vi "Autonomous Independent.vi"   [LabVIEW 2011]
doc: "This VI is called when autonomous begins, and will automatically be terminated when autonomous ends. You can carry out timed or sensor driven robot movement independently without needing to return to the caller."
uses:
  Robot Global Data.vi
types:
  T1 = typedef "WPI_MotorControlDeviceRef.ctl" = cluster{"DeviceStatus":errorcluster, "Type":enum16{"PWM", "CAN"}, "PWM":cluster{"Digital Module":T2, "PWM Channel":T3, "DeadBand":T4}, "CAN":cluster{"Device Number":u8, "Control Mode":T5, "Semaphore":T6, "Max Vout":dbl}, "Invert":bool, "TransformRef":T7, "InvTransformRef":T7}
  T2 = typedef "FPGA_TypedefDigitalModule.ctl" = enum16{"Digital Module 1", "Digital Module 2"}
  T3 = typedef "FPGA_DIOPWMChannel.ctl" = enum8{"PWM 1", "PWM 2", "PWM 3", "PWM 4", "PWM 5", "PWM 6", "PWM 7", "PWM 8", "PWM 9", "PWM 10", "Invalid"}
  T4 = typedef "WPI_PWMDeadband.ctl" = cluster{"Name":string, "maxPositivePwm":i32, "minPositivePwm":i32, "centerPwm":i32, "maxNegativePwm":i32, "minNegativePwm":i32, "angularRange":u16}
  T5 = typedef "WPI_CANJaguar_ControlMode.ctl" = enum8{"Percent VBus", "Current", "Speed", "Position", "Voltage"}
  T6 = typedef "Semaphore RefNum" = refnum<k1>
  T7 = typedef "WPI_PWMTransform_ConPane.ctl" = refnum<vi>
  T8 = typedef "WPI_ServoDeviceRef.ctl" = cluster{"DeviceStatus":errorcluster, "Digital Module":T2, "PWM Channel":T3, "DeadBand":T4}
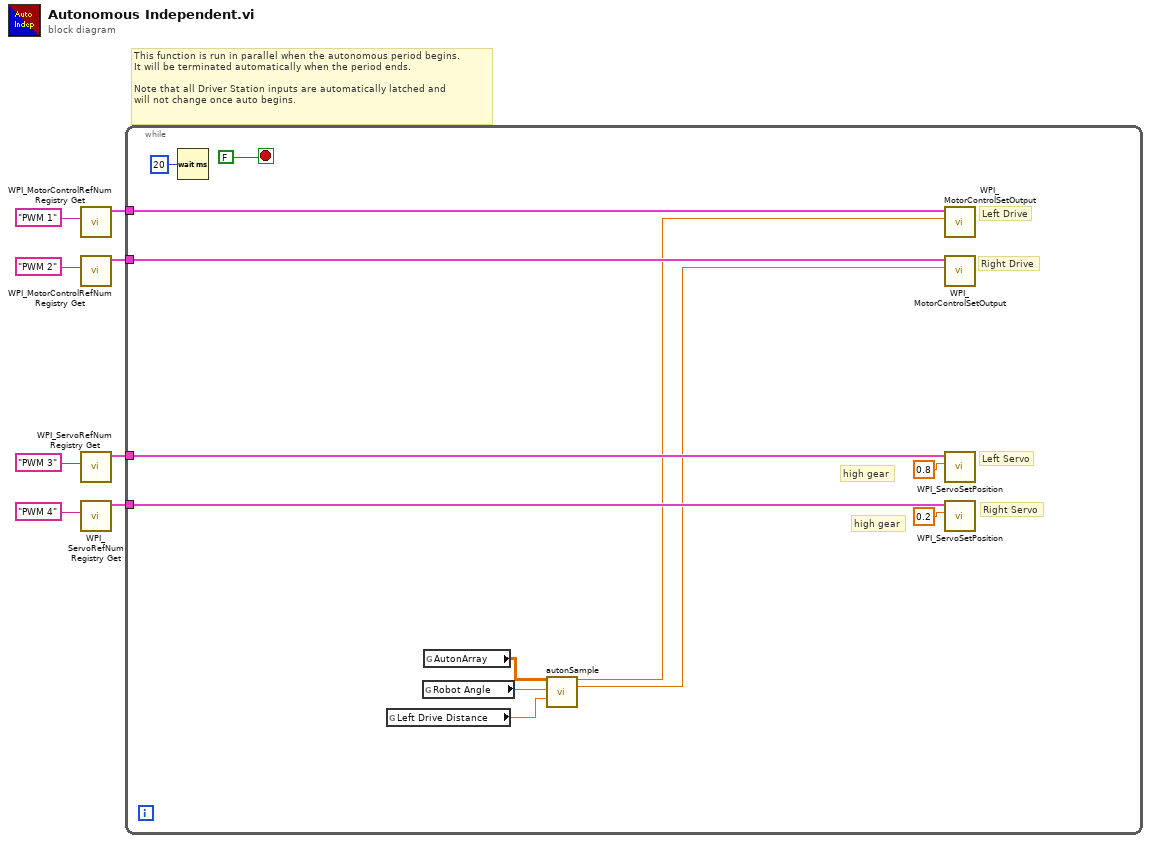
[diagram p0: block diagram]
diagram:
  # "This function is run in parallel when the autonomous period begins.\nIt will be terminated automatically when the period ends.\n\nNote that all Driver Station inputs are automatically latched and\nwill not change once auto begins."
  n1 = call <vilib>:"WPI_MotorControlRefNum Registry Get.vi"("refnum name"="PWM 1") -> ("MotorControlDevRef"=w4:T1)  [unwired: 1 in, 9 out]
  n2 = call <vilib>:"WPI_MotorControlRefNum Registry Get.vi"("refnum name"="PWM 2") -> ("MotorControlDevRef"=w3:T1)  [unwired: 1 in, 9 out]
  n3 = call <vilib>:"WPI_ServoRefNum Registry Get.vi"("refnum name"="PWM 3") -> ("ServoDeviceRef"=w2:T8)  [unwired: 1 in, 9 out]
  n4 = call <vilib>:"WPI_ServoRefNum Registry Get.vi"("refnum name"="PWM 4") -> ("ServoDeviceRef"=w1:T8)  [unwired: 1 in, 9 out]
  n5 = while {
    tunnel: w4 -> [w19]
    tunnel: w3 -> [w18]
    tunnel: w2 -> [w16]
    tunnel: w1 -> [w17]
    stop <- FALSE stop-if-true
    # "high gear"
    # "high gear"
    # "Right Servo"
    # "Left Servo"
    # "Right Drive"
    # "Left Drive"
    n6 = Wait (ms)(milliseconds to wait=u32 20) -> ()  [unwired: 1 out]
    n7 = global read "Robot Global Data.vi" "Left Drive Distance"() -> (w14:dbl)
    n8 = global read "Robot Global Data.vi" "Robot Angle"() -> (w15:dbl)
    n9 = global read "Robot Global Data.vi" "AutonArray"() -> (w13:dbl[][])
    n10 = call "autonSample.vi"("Auton Array"=w13, "MeasuredHeading"=w15, "EncoderDistance"=w14) -> ("Left Drive"=w12:dbl, "Right Drive"=w11:dbl)  [unwired: 11 out]
    n11 = call <vilib>:"WPI_MotorControlSetOutput.vi"("Output"=w12, "MotorControlDevRef"=w19) -> ()  [unwired: 3 in, 7 out]
    n12 = call <vilib>:"WPI_MotorControlSetOutput.vi"("Output"=w11, "MotorControlDevRef"=w18) -> ()  [unwired: 3 in, 7 out]
    n13 = call <vilib>:"WPI_ServoSetPosition.vi"("Position"=0.8, "ServoDeviceRef"=w16) -> ()  [unwired: 1 in, 9 out]
    n14 = call <vilib>:"WPI_ServoSetPosition.vi"("Position"=0.2, "ServoDeviceRef"=w17) -> ()  [unwired: 1 in, 9 out]
  }
